vi "detector_get_counts_1d_dbl.vi"(8 "error in (no error)":errorcluster, 11 "picoharp in":refnum<class "picoharp.lvclass">) -> (0 "error out":errorcluster, 2 "counts":dbl[](array[numeric]), 3 "picoharp out":refnum<class "picoharp.lvclass">)   [LabVIEW 2015, in "picoharp.lvclass"]
uses:
  picoharp.lvclass
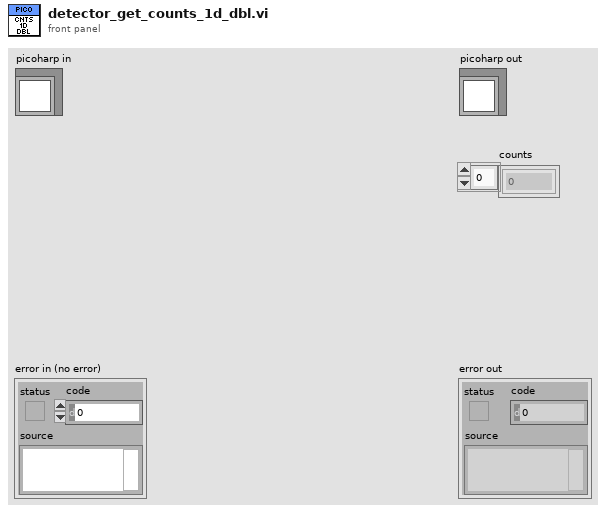
[diagram p1: front panel]
types:
  T1 = typedef "hydraharp_count_rates.ctl" = cluster{"channel_rates":i32[], "sync_rate":i32}
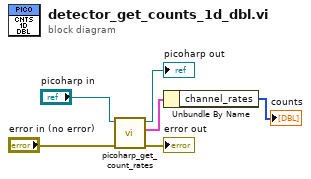
[diagram p0: block diagram]
diagram:
  n1 = call "picoharp_get_count_rates.vi"("error in (no error)"="error in (no error)", "hydraharp in"="picoharp in") -> ("error out"=→"error out":errorcluster, "count_rates"=w2:T1, "hydraharp out"=→"picoharp out":refnum<class "picoharp.lvclass">)  [unwired: 7 in]
  n2 = Unbundle By Name(w2) -> ("channel_rates"=→"counts":i32[])
